vi "RegisterImageRoutedMessage_Parse.vi"(8 "error in (no error)":errorcluster, 9 "message":variant) -> (0 "error out":errorcluster, 2 "RegisterImageRoutedMessage data":T1)   [LabVIEW 2017, in "IrDataEventCreator.lvlib"]
uses:
  <vilib>/addons/InsightCM/Devices/Shared/Ir/IrDataEventCreator/IrDataEventCreator.lvlib
  <vilib>/addons/InsightCM/Devices/Shared/Ir/IrDataEventCreator/controls/RegisterImageRoutedMessage.ctl
  <vilib>/addons/InsightCM/Devices/Shared/Ir/IrDataEventCreator/controls/Registry_Image.ctl
  <vilib>/addons/InsightCM/MessageBus/Base/controls/KeyValuePair.ctl
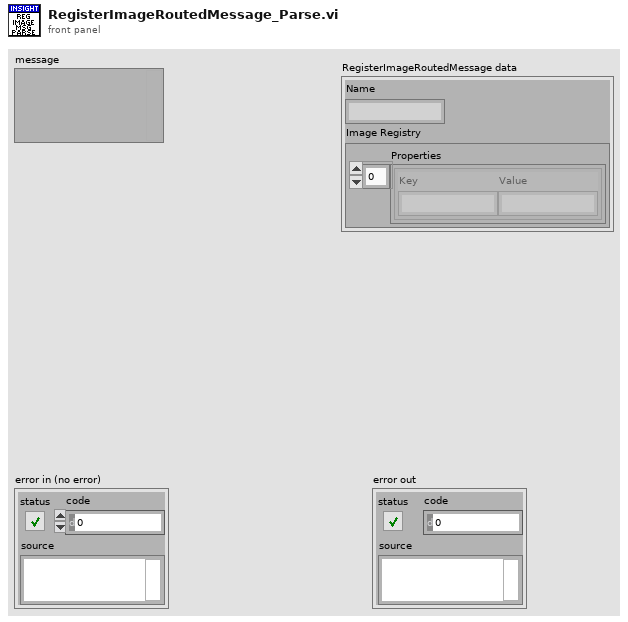
[diagram p1: front panel]
types:
  T1 = typedef "IrDataEventCreator.lvlib/RegisterImageRoutedMessage.ctl" = cluster{"Name":string, "Image Registry":T2}
  T2 = typedef "IrDataEventCreator.lvlib/Registry_Image.ctl" = cluster{"Properties":T3[]}
  T3 = typedef "KeyValuePair.ctl" = cluster{"Key":string, "Value":string}
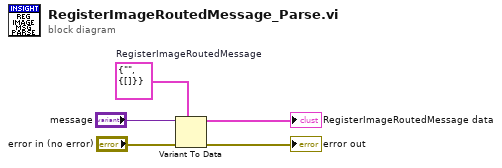
[diagram p0: block diagram]
diagram:
  w2 = T1 {"Name"="", "Image Registry"={"Properties"=[]}}  # RegisterImageRoutedMessage
  n1 = Variant To Data(error in="error in (no error)", type=w2, Variant="message") -> (data=→"RegisterImageRoutedMessage data":T1, error out=→"error out":errorcluster)
